vi "CurrentServoConnectionStatus.vi"(8 "New Servo Connection Status":T1, 11 "Operation":T2) -> (3 "Current Servo Connection Status":T1)   [LabVIEW 2024]
uses:
  DataTypes/OperationTypeForFunctionalGlobalVariable.ctl
  DataTypes/ServoConnectionStatus.ctl
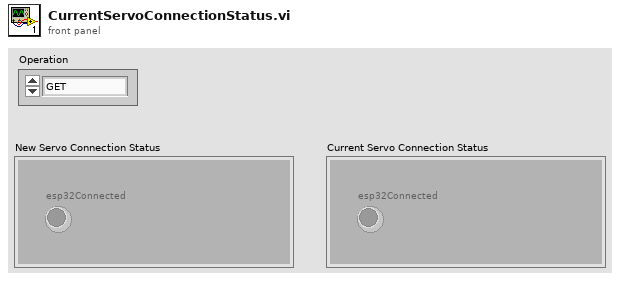
[diagram p1: front panel]
types:
  T1 = typedef "ServoConnectionStatus.ctl" = cluster{"esp32Connected":bool}
  T2 = typedef "OperationTypeForFunctionalGlobalVariable.ctl" = enum16{"GET", "SET"}
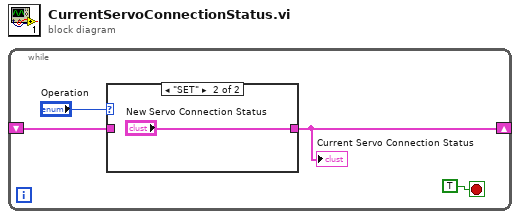
[diagram p0: block diagram]
diagram:
  n1 = while {
    shift-right: [w1] -> _
    shift-left: _ -> [w3]
    stop <- TRUE stop-if-true
    n2 = case shown="\"SET\"" "Operation" {
      tunnel: w3 -> [w5 _]
      tunnel: [w5 "New Servo Connection Status"] -> w1
      frame "GET", Default {
      }
      frame "SET" {
      }
    }
    "Current Servo Connection Status" <- w1
  }
